vi "build test.vi"() -> ()   [LabVIEW 2010]
panel:
  in  "App.Kind":T1(ring)
  in  "relative path (.)":path=path ""
  out "current VI's path + relative path":path
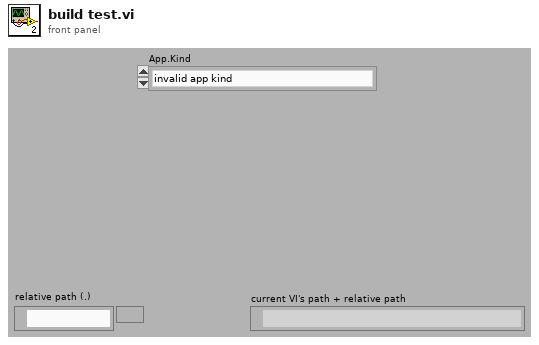
[diagram p1: front panel]
types:
  T1 = enum32{"invalid app kind", "Development System", "Run Time System", "Student Edition", "Embedded LabVIEW", "Evaluation", "Custom"}
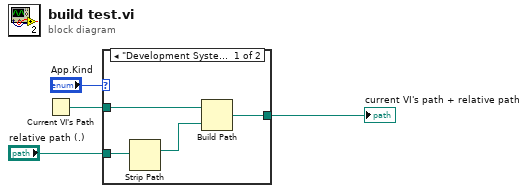
[diagram p0: block diagram]
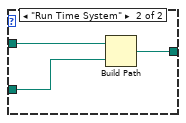
[diagram p2: hidden frame]
diagram:
  n1 = Current VI's Path() -> (path=w4:path)
  n2 = case shown="\"Development System\", Default" "App.Kind" {
    tunnel: [w8 w9] -> w2
    tunnel: w4 -> [w7 w11]
    tunnel: "relative path (.)" -> [w6 w10]
    frame "Development System", Default {
      n3 = Strip Path(path=w6) -> (stripped path=w5:path)  [unwired: 1 out]
      n4 = Build Path(base path=w7, name or relative path=w5) -> (appended path=w8:path)
    }
    frame "Run Time System" {
      n5 = Build Path(base path=w11, name or relative path=w10) -> (appended path=w9:path)
    }
  }
  "current VI's path + relative path" <- w2
